vi "Parse Sensor Status.vi"(7 "Aircraft System Status":T1 {"Communication Drop Rate (%)" scale=0.0..100.0; "Battery Remaining (%)" scale=0.0..100.0; "CPU Load (%)" scale=0.0..100.0}, 9 "Healthy":bool[](array[boolean]), 10 "Enabled":bool[](array[boolean]), 11 "Present":bool[](array[boolean])) -> (3 "Aircraft System Status Out":T1 {"Communication Drop Rate (%)" scale=0.0..100.0; "Battery Remaining (%)" scale=0.0..100.0; "CPU Load (%)" scale=0.0..100.0})   [LabVIEW 2014]
uses:
  Aircraft Information/Controls/Aircraft Sensor Status Data.ctl
  GUI Design/Indicators/Sensor Status LED CLuster.ctl
  GUI Design/Indicators/Status LED.ctl
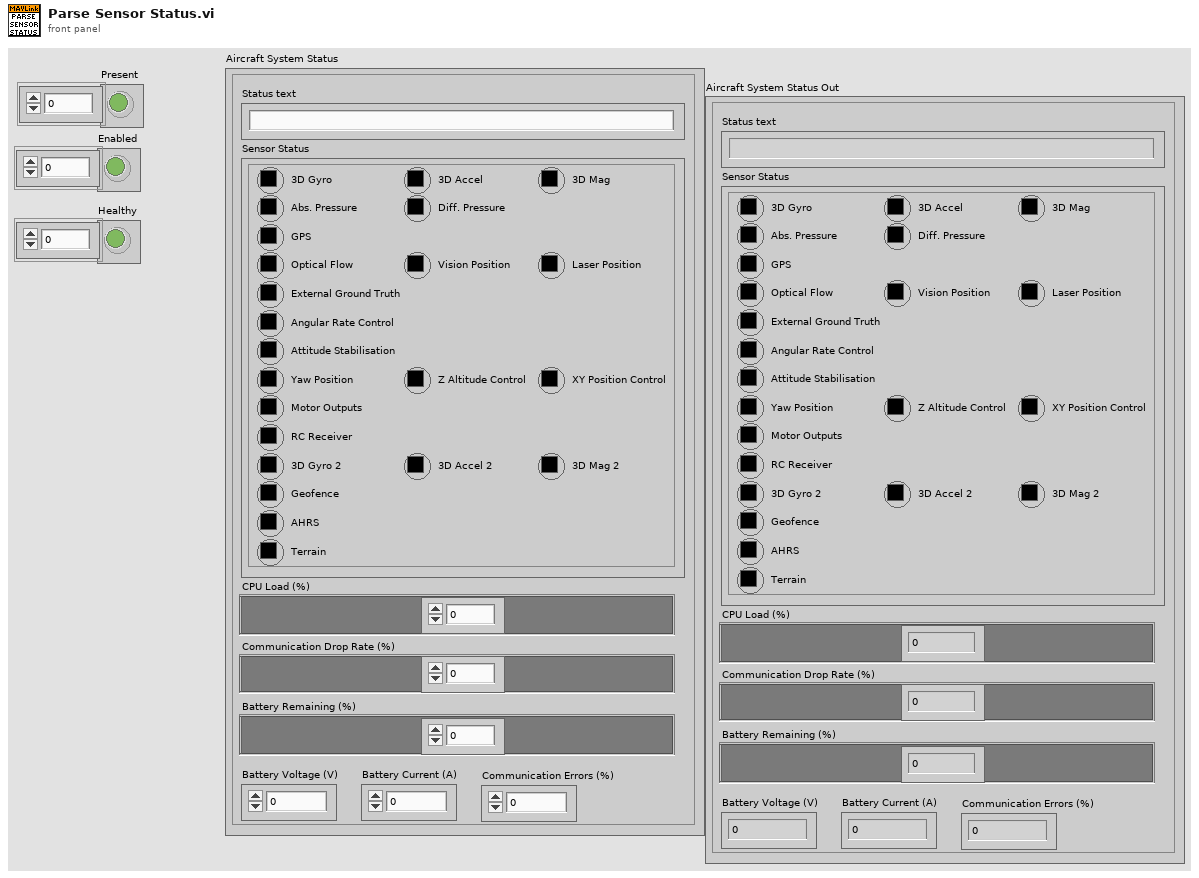
[diagram p1: front panel]
types:
  T1 = typedef "Aircraft Sensor Status Data.ctl" = cluster{"Sensor Status":T2, "CPU Load (%)":dbl, "Battery Voltage (V)":dbl, "Battery Current (A)":dbl, "Battery Remaining (%)":dbl, "Communication Drop Rate (%)":dbl, "Communication Errors (%)":dbl, "Status text":string}
  T2 = typedef "Sensor Status LED CLuster.ctl" = cluster{"3D Gyro":u32, "3D Accel":u32, "3D Mag":u32, "Abs. Pressure":u32, "Diff. Pressure":u32, "GPS":T3, "Optical Flow":u32, "Vision Position":u32, "Laser Position":u32, "External Ground Truth":u32, "Angular Rate Control":u32, "Attitude Stabilisation":u32, "Yaw Position":u32, "Z Altitude Control":u32, "XY Position Control":u32, "Motor Outputs":u32, "RC Receiver":u32, "3D Gyro 2":u32, "3D Accel 2":u32, "3D Mag 2":u32, "Geofence":u32, "AHRS":u32, "Terrain":u32}
  T3 = typedef "Status LED.ctl" = u32
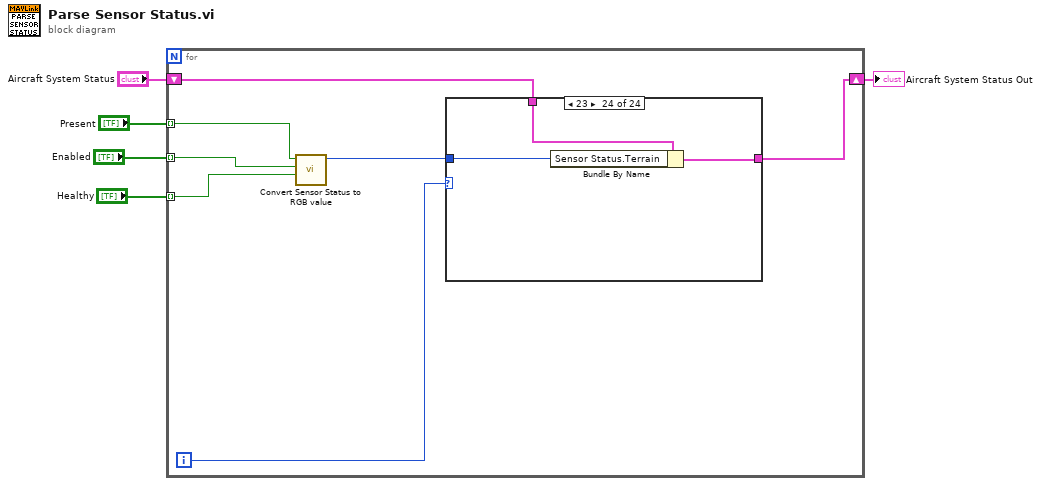
[diagram p0: block diagram]
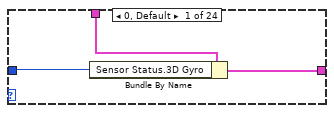
[diagram p2: hidden frame]
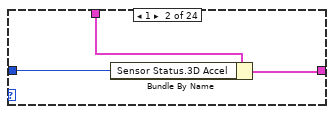
[diagram p3: hidden frame]
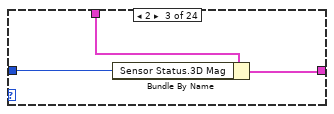
[diagram p4: hidden frame]
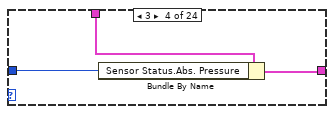
[diagram p5: hidden frame]
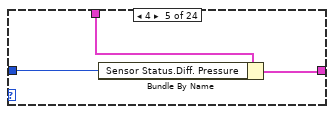
[diagram p6: hidden frame]
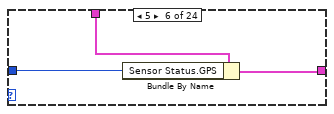
[diagram p7: hidden frame]
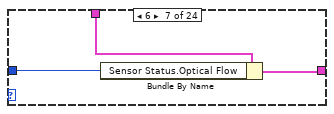
[diagram p8: hidden frame]
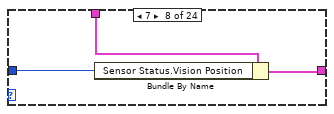
[diagram p9: hidden frame]
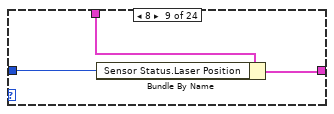
[diagram p10: hidden frame]
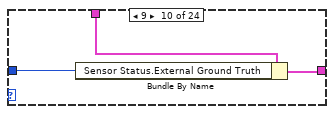
[diagram p11: hidden frame]
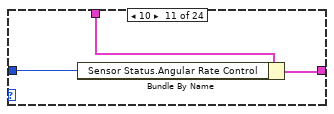
[diagram p12: hidden frame]
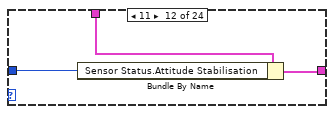
[diagram p13: hidden frame]
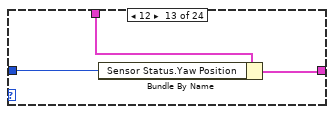
[diagram p14: hidden frame]
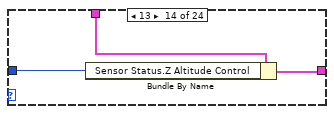
[diagram p15: hidden frame]
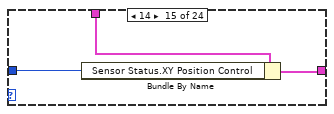
[diagram p16: hidden frame]
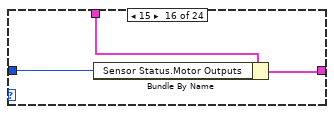
[diagram p17: hidden frame]
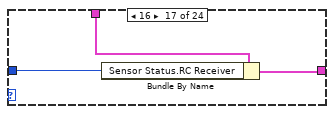
[diagram p18: hidden frame]
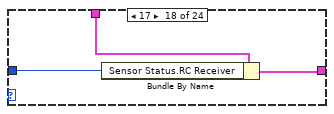
[diagram p19: hidden frame]
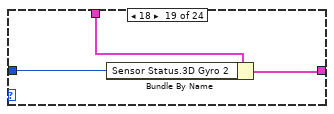
[diagram p20: hidden frame]
diagram:
  n1 = for {
    tunnel: "Present" -> [w12] mode=indexing
    tunnel: "Enabled" -> [w11] mode=indexing
    tunnel: "Healthy" -> [w10] mode=indexing
    shift-right: [w7] -> w1
    shift-left: "Aircraft System Status" -> [w8]
    i -> [w9]
    n2 = call "Convert Sensor Status to RGB value.vi"("Sensor Healthy"=w10, "Sensor Enabled"=w11, "Sensor Present"=w12) -> ("Sensor Status"=w6:u32)  [unwired: 8 in]
    n3 = case shown="23" w9 {
      tunnel: w8 -> [w15 w18 w21 w24 w27 w30 w33 w36 w39 w42 w45 w48 w51 w54 w57 w60 w63 w66 w69 w72 w75 w78 w81 w84]
      tunnel: [w14 w17 w20 w23 w26 w29 w32 w35 w38 w41 w44 w47 w50 w53 w56 w59 w62 w65 w68 w71 w74 w77 w80 w83] -> w7
      tunnel: w6 -> [w13 w16 w19 w22 w25 w28 w31 w34 w37 w40 w43 w46 w49 w52 w55 w58 w61 w64 w67 w70 w73 w76 w79 w82]
      frame 0, Default {
        n4 = Bundle By Name(cluster=w15, "Sensor Status.3D Gyro"=w13) -> (w14:T1)
      }
      frame 1 {
        n5 = Bundle By Name(cluster=w18, "Sensor Status.3D Accel"=w16) -> (w17:T1)
      }
      frame 2 {
        n6 = Bundle By Name(cluster=w21, "Sensor Status.3D Mag"=w19) -> (w20:T1)
      }
      frame 3 {
        n7 = Bundle By Name(cluster=w24, "Sensor Status.Abs. Pressure"=w22) -> (w23:T1)
      }
      frame 4 {
        n8 = Bundle By Name(cluster=w27, "Sensor Status.Diff. Pressure"=w25) -> (w26:T1)
      }
      frame 5 {
        n9 = Bundle By Name(cluster=w30, "Sensor Status.GPS"=w28) -> (w29:T1)
      }
      frame 6 {
        n10 = Bundle By Name(cluster=w33, "Sensor Status.Optical Flow"=w31) -> (w32:T1)
      }
      frame 7 {
        n11 = Bundle By Name(cluster=w36, "Sensor Status.Vision Position"=w34) -> (w35:T1)
      }
      frame 8 {
        n12 = Bundle By Name(cluster=w39, "Sensor Status.Laser Position"=w37) -> (w38:T1)
      }
      frame 9 {
        n13 = Bundle By Name(cluster=w42, "Sensor Status.External Ground Truth"=w40) -> (w41:T1)
      }
      frame 10 {
        n14 = Bundle By Name(cluster=w45, "Sensor Status.Angular Rate Control"=w43) -> (w44:T1)
      }
      frame 11 {
        n15 = Bundle By Name(cluster=w48, "Sensor Status.Attitude Stabilisation"=w46) -> (w47:T1)
      }
      frame 12 {
        n16 = Bundle By Name(cluster=w51, "Sensor Status.Yaw Position"=w49) -> (w50:T1)
      }
      frame 13 {
        n17 = Bundle By Name(cluster=w54, "Sensor Status.Z Altitude Control"=w52) -> (w53:T1)
      }
      frame 14 {
        n18 = Bundle By Name(cluster=w57, "Sensor Status.XY Position Control"=w55) -> (w56:T1)
      }
      frame 15 {
        n19 = Bundle By Name(cluster=w60, "Sensor Status.Motor Outputs"=w58) -> (w59:T1)
      }
      frame 16 {
        n20 = Bundle By Name(cluster=w63, "Sensor Status.RC Receiver"=w61) -> (w62:T1)
      }
      frame 17 {
        n21 = Bundle By Name(cluster=w66, "Sensor Status.RC Receiver"=w64) -> (w65:T1)
      }
      frame 18 {
        n22 = Bundle By Name(cluster=w69, "Sensor Status.3D Gyro 2"=w67) -> (w68:T1)
      }
      frame 19 {
        n23 = Bundle By Name(cluster=w72, "Sensor Status.3D Accel 2"=w70) -> (w71:T1)
      }
      frame 20 {
        n24 = Bundle By Name(cluster=w75, "Sensor Status.3D Mag 2"=w73) -> (w74:T1)
      }
      frame 21 {
        n25 = Bundle By Name(cluster=w78, "Sensor Status.Geofence"=w76) -> (w77:T1)
      }
      frame 22 {
        n26 = Bundle By Name(cluster=w81, "Sensor Status.AHRS"=w79) -> (w80:T1)
      }
      frame 23 {
        n27 = Bundle By Name(cluster=w84, "Sensor Status.Terrain"=w82) -> (w83:T1)
      }
    }
  }
  "Aircraft System Status Out" <- w1
